vi "CNR initial TR radius.vi"(8 "error in":errorcluster, 10 "g":dbl[](array[numeric]), 11 "H":T1) -> (0 "error out":errorcluster, 3 "initial TR radius":dbl)   [LabVIEW 2014, in "NI_Gmath.lvlib"]
uses:
  NI_Gmath.lvlib
  RealMatrix.ctl
  Real Dot Product.vi
  A x Vector.vi
  NI_AALBase.lvlib
  NI_Matrix.lvlib
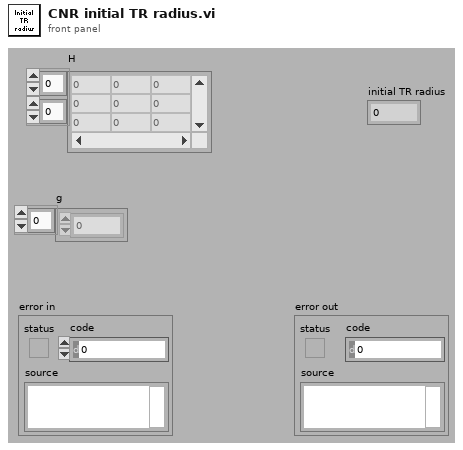
[diagram p1: front panel]
types:
  T1 = typedef "NI_Matrix.lvlib/RealMatrix.ctl" = dbl[][]
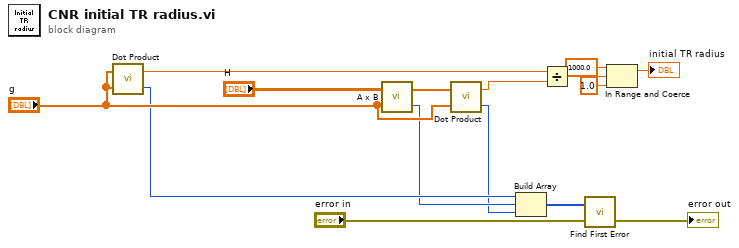
[diagram p0: block diagram]
diagram:
  n1 = call-poly "Dot Product.vi"("Y Vector"="g", "X Vector"="g") -> ("error"=w6:i32, "X * Y"=w12:dbl)
  n2 = call-poly "A x B.vi"("Vector"="g", "A"="H") -> ("error"=w5:i32, "A x Vector"=w14:dbl[])
  n3 = call-poly "Dot Product.vi"("Y Vector"="g", "X Vector"=w14) -> ("error"=w4:i32, "X * Y"=w11:dbl)
  n4 = Build Array(w6, w5, w4) -> (w3:i32[])
  n5 = Divide(x=w12, y=w11) -> (x/y=w10:dbl)
  n6 = call "Find First Error.vi"("error in (no error)"="error in", "error codes"=w3) -> ("error out"=→"error out":errorcluster)  [unwired: 2 in, 1 out]
  n7 = In Range and Coerce(upper limit=1000.0, x=w10, lower limit=1.0) -> (coerced(x)=→"initial TR radius":dbl)  [unwired: 1 out]
